vi "aggregation-lifetime-management.vi"(8 "error in (no error)":errorcluster) -> (0 "error out":errorcluster)   [LabVIEW 2021]
uses:
  src/SMO/SMO.lvclass
  <vilib>/addons/_JKI Toolkits/Caraya/classes/Test/Test.lvclass
  <vilib>/addons/_JKI Toolkits/Caraya/classes/Assert/Assert.lvclass
panel:
  # "<< Error 1556 illustrates a bug with version 1.1.7.31 \n\n(Essentially because B is destroyed by top-level before A is stopped, and A depends on B that no longer exists on stopping... this error should be handled by framework. Reverse the launching order to demonstrate bug is lifetime-related)"
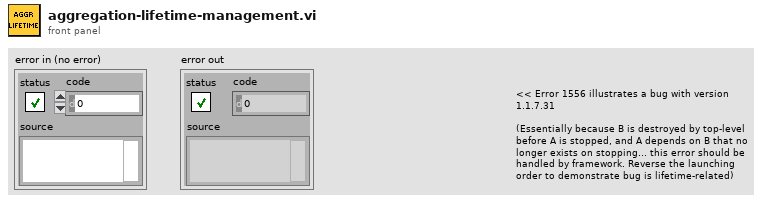
[diagram p1: front panel]
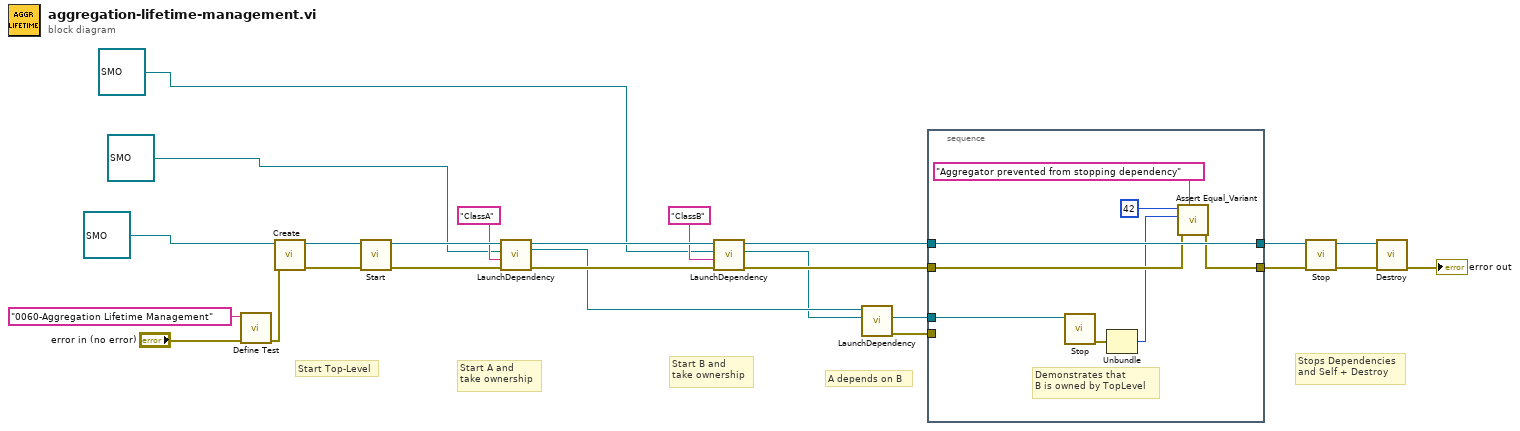
[diagram p0: block diagram]
diagram:
  # "Stops Dependencies\nand Self + Destroy"
  # "A depends on B"
  # "Start B and\ntake ownership"
  # "Start A and\ntake ownership"
  # "Start Top-Level"
  n1 = call <vilib>:"Define Test.vi"("error in (no error)"="error in (no error)", "Label (VI Title)"="0060-Aggregation Lifetime Management") -> ("error out"=w4:errorcluster)  [unwired: 9 in]
  n2 = call "Create.vi"("error in (no error)"=w4, "SMO"=refnum<class "SMO.lvclass"> refnum ("Dependency Type")) -> ("error out"=w19:errorcluster, "SMO out"=w25:refnum<class "SMO.lvclass">)  [unwired: 7 in, 1 out]
  n3 = call "Start.vi"("error in (no error)"=w19, "SMO"=w25) -> ("error out"=w20:errorcluster, "SMO out"=w24:refnum<class "SMO.lvclass">)  [unwired: 8 in]
  n4 = call "LaunchDependency.vi"("error in (no error)"=w20, "Dependency Name"="ClassA", "Dependency Type"=refnum<class "SMO.lvclass"> refnum, "SMO in"=w24) -> ("error out"=w18:errorcluster, "Dependency Reference"=w9:refnum<class "SMO.lvclass">, "SMO out"=w22:refnum<class "SMO.lvclass">)  [unwired: 4 in, 1 out]
  n5 = call "LaunchDependency.vi"("error in (no error)"=w18, "Dependency Name"="ClassB", "Dependency Type"=refnum<class "SMO.lvclass"> refnum, "SMO in"=w22) -> ("error out"=w15:errorcluster, "Dependency Reference"=w8:refnum<class "SMO.lvclass">, "SMO out"=w16:refnum<class "SMO.lvclass">)  [unwired: 4 in, 1 out]
  n6 = call "LaunchDependency.vi"("Dependency Type"=w8, "SMO in"=w9) -> ("error out"=w17:errorcluster, "Dependency Reference"=w14:refnum<class "SMO.lvclass">)  [unwired: 6 in, 2 out]
  n7 = stacked-sequence {
    tunnel: w17 -> [_]
    tunnel: w16 -> [w31]
    tunnel: w15 -> [w30]
    tunnel: w14 -> [w33]
    tunnel: [w31] -> w13
    tunnel: [w29] -> w12
    frame #0 {
      # "Demonstrates that\nB is owned by TopLevel"
      n8 = call "Stop.vi"("SMO"=w33) -> ("error out"=w32:errorcluster)  [unwired: 9 in, 1 out]
      n9 = Unbundle(w32) -> ("code"=w28:i32)  [unwired: 2 out]
      n10 = call <vilib>:"Assert Equal_Variant.vi"("Label"="Aggregator prevented from stopping dependency" ("Dependency Name"), "error in (no error)"=w30, "Y"=w28, "X"=42 ("y")) -> ("error out"=w29:errorcluster)  [unwired: 7 in]
    }
  }
  n11 = call "Stop.vi"("error in (no error)"=w12, "SMO"=w13) -> ("error out"=w10:errorcluster, "SMO out"=w11:refnum<class "SMO.lvclass">)  [unwired: 8 in]
  n12 = call "Destroy.vi"("error in (no error)"=w10, "SMO"=w11) -> ("error out"=→"error out":errorcluster)  [unwired: 9 in]
